vi "StringArrayVariableParse.vi"(8 "error in":errorcluster, 9 "Info":T1, 10 "in":string, 11 "dictionary":T2) -> (0 "error out":errorcluster, 1 "after match":string, 2 "ValueArray":string[](array[string]), 3 "Find?":bool, 5 "before match":string)   [LabVIEW 2018]
uses:
  <userlib>/_OpenG.lib/dictionary/dictionary.llb/Dictionary Object RefNum__ogtk.ctl
  <userlib>/_OpenG.lib/dictionary/dictionary.llb/Dictionary Object RefNum - Enum__ogtk.ctl
  <vilib>/regexp/Match Regular Expression.xnode
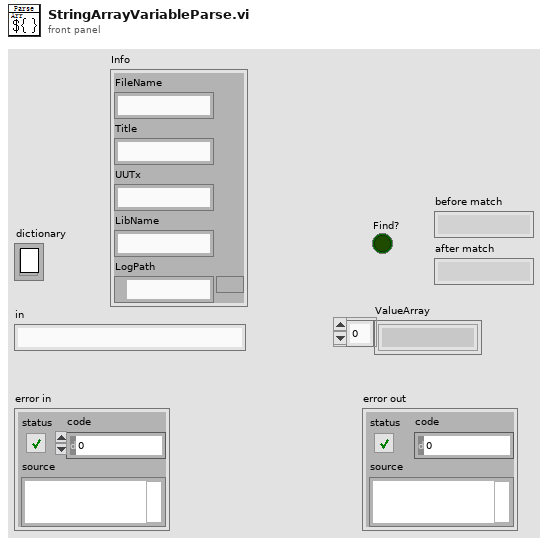
[diagram p1: front panel]
types:
  T1 = cluster{"FileName":string, "Title":string, "UUTx":string, "LibName":string, "LogPath":path}
  T2 = typedef "Dictionary Object RefNum__ogtk.ctl" = refnum<k1>
  T3 = cluster{"Describe":string, "ValueArray":string[]}
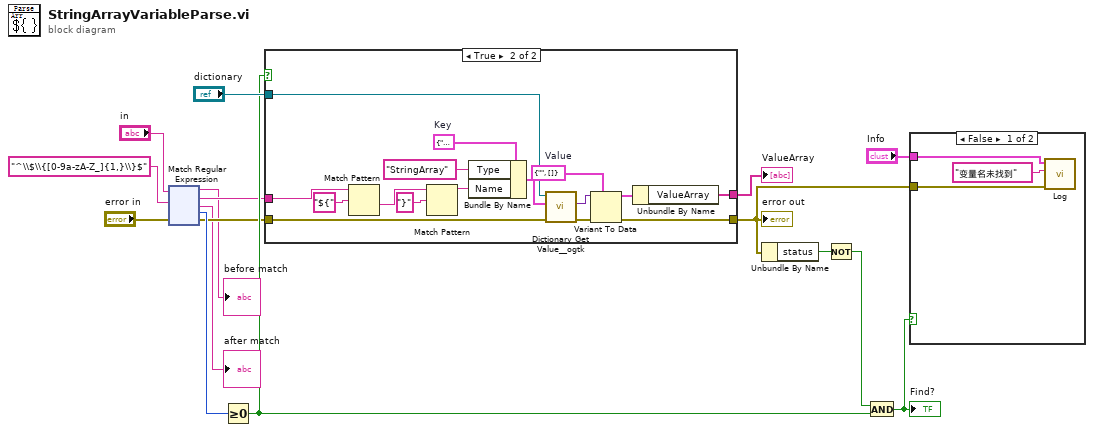
[diagram p0: block diagram]
diagram:
  n1 = xnode "Match Regular Expression"("input string"="in", "regular expression"="^\\$\\{[0-9a-zA-Z_]{1,}\\}$", "error in"="error in") -> ("before match"=→"before match":string, "whole match"=w10:string, "after match"=→"after match":string, "offset past match"=w12:i32, "error out"=w7:errorcluster)  [unwired: 3 in]
  n2 = Greater Or Equal To 0?(x=w12) -> (x >= 0?=w11:bool)
  n3 = case shown="True" w11 {
    tunnel: [_ w19] -> w6
    tunnel: "dictionary" -> [_ w31]
    tunnel: w10 -> [_ w27]
    tunnel: w7 -> [w17 w26]
    tunnel: [w17 w25] -> w1
    frame False {
    }
    frame True {
      w21 = T3 {"Describe"="", "ValueArray"=[]}  # Value
      w24 = cluster{"Type":string, "Name":string} {"Type"="", "Name"=""}  # Key
      n4 = Match Pattern(string=w27, regular expression="${") -> (after substring=w30:string)  [unwired: 1 in, 3 out]
      n5 = Match Pattern(string=w30, regular expression="}") -> (before substring=w23:string)  [unwired: 1 in, 3 out]
      n6 = Bundle By Name(cluster=w24, "Type"="StringArray", "Name"=w23) -> (w22:cluster{"Type":string, "Name":string})
      n7 = call <userlib>:"Dictionary Get Value__ogtk.vi"("error in"=w26, "key"=w22, "dictionary"=w31) -> ("error out"=w33:errorcluster, "value"=w32:variant)  [unwired: 5 in, 2 out]
      n8 = Variant To Data(error in=w33, type=w21, Variant=w32) -> (data=w20:T3, error out=w25:errorcluster)
      n9 = Unbundle By Name(w20) -> ("ValueArray"=w19:string[])
    }
  }
  "error out" <- w1
  "ValueArray" <- w6
  n10 = Unbundle By Name(w1) -> ("status"=w9:bool)
  n11 = Not(x=w9) -> (.not. x?=w8:bool)
  n12 = And(x=w8, y=w11) -> (x .and. y?=w2:bool)
  "Find?" <- w2
  n13 = case shown="False" w2 {
    tunnel: "Info" -> [w36 _]
    tunnel: w1 -> [w35 _]
    frame False {
      n14 = call "Log.vi"("error in"=w35, "LogIn"="变量名未找到", "Info"=w36) -> ()  [unwired: 9 in]
    }
    frame True {
    }
  }
